vi "Variable list Tool digital.vi"() -> (6 "Variant":variant, 10 "Array":T1[](array[typedef]))   [LabVIEW 2011]
uses:
  Measurments Handling/Fixed Digital Channel Definition.ctl
  Measurments Handling/Update frequensies.ctl
  Measurments Handling/Channel catagory Enum.ctl
  Variable List Tool Digital.ctl
  Measurments Handling/Common/Variable List Common Digital.ctl
  <vilib>/Utility/VariantDataType/GetNumericInfo.vi
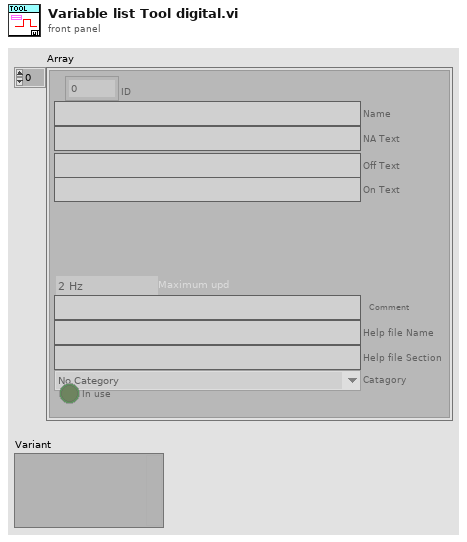
[diagram p1: front panel]
types:
  T1 = typedef "Fixed Digital Channel Definition.ctl" = cluster{"ID":u16, "Name":string, "NA Text":string, "Off Text":string, "On Text":string, "Maximum upd":T2, "Comment":string, "Help file Name":string, "Help file Section ":string, "Catagory":T3, "In use":bool}
  T2 = typedef "Update frequensies.ctl" = enum16{"2 Hz", "1 Hz", "0.1 Hz"}
  T3 = typedef "Channel catagory Enum.ctl" = enum16{"No Category", "Power", "Temperature", "Pressure"}
  T4 = typedef "Variable List Common Digital.ctl" = enum16{"PCP Connected", "PCP PC Control", "HV PSU connected", "HV PSU HV Active", "Modem Connected", "Tool Connected", "CanBus interface"}
  T5 = typedef "Variable List Tool Digital.ctl" = enum16{"Tool Error Controller", "Tool Stopped Controller", "Tool Relay 1", "Tool Relay 2", "Tool Both Relays", "Tool node Pressure 1", "Tool Error Pressure 1", "Tool Stopped Pressure 1", "Tool node Pressure 2", "Tool Error Pressure 2", "Tool Stopped Pressure 2", "Tool node Solenoid", "Tool Error Solenoid", "Tool Stopped Solenoid", "Tool Solenoid 1", "Tool Solenoid 2", "Tool Solenoid 3", "Tool node PSU", "Tool Error PSU", "Tool Stopped PSU", "Upper Tension Sub", "Tool Error Upper Tension Sub", "Tool Stopped Upper Tension Sub", "Lower Tension Sub", "Tool Error Lower Tension Sub", "Tool Stopped Lower Tension Sub", "Stroke Target seeking", "Stroke Moving Out", "Stroke Moving Inn", "Stroke valves set for Out", "Stroke valves set for In", "Stroke In (force)", "Stroke Out (force)", "Stroke Force decreasing(in)", "Stroke Force decreasing(out)", "Stroke Force change not correct", "Stroke SLIPS established P1", "Stroke SLIPS established P2", "Stroke SLIPS established", "Stroke Pressure Monitor Ongoing", "Stroke Pressure Monitor Ending ", "Tool Stroke enable Valve", "Tool Stroke direction Valve", "Tool Anchor Valve", "Stroker Var19 - Reserved", "Stroker Var20 - Reserved", "Stroker Var21 - Reserved", "Stroker Var22 - Reserved", "Stroker Var23 - Reserved", "Stroker Var24 - Reserved", "Tractor Var1 - Reserved", "Tractor Var2 - Reserved", "Tractor Var3 - Reserved", "Tractor Var4 - Reserved", "Tractor Var5 - Reserved", "Tractor Var6 - Reserved", "Tractor Var7 - Reserved", "Tractor Var8 - Reserved", "Oil filling mode", "Mill Bit Direction", "Position control", "Anchor", "Driller Var5 - Reserved", "Driller Var6 - Reserved", "Driller Var7 - Reserved", "Driller Var8 - Reserved"}
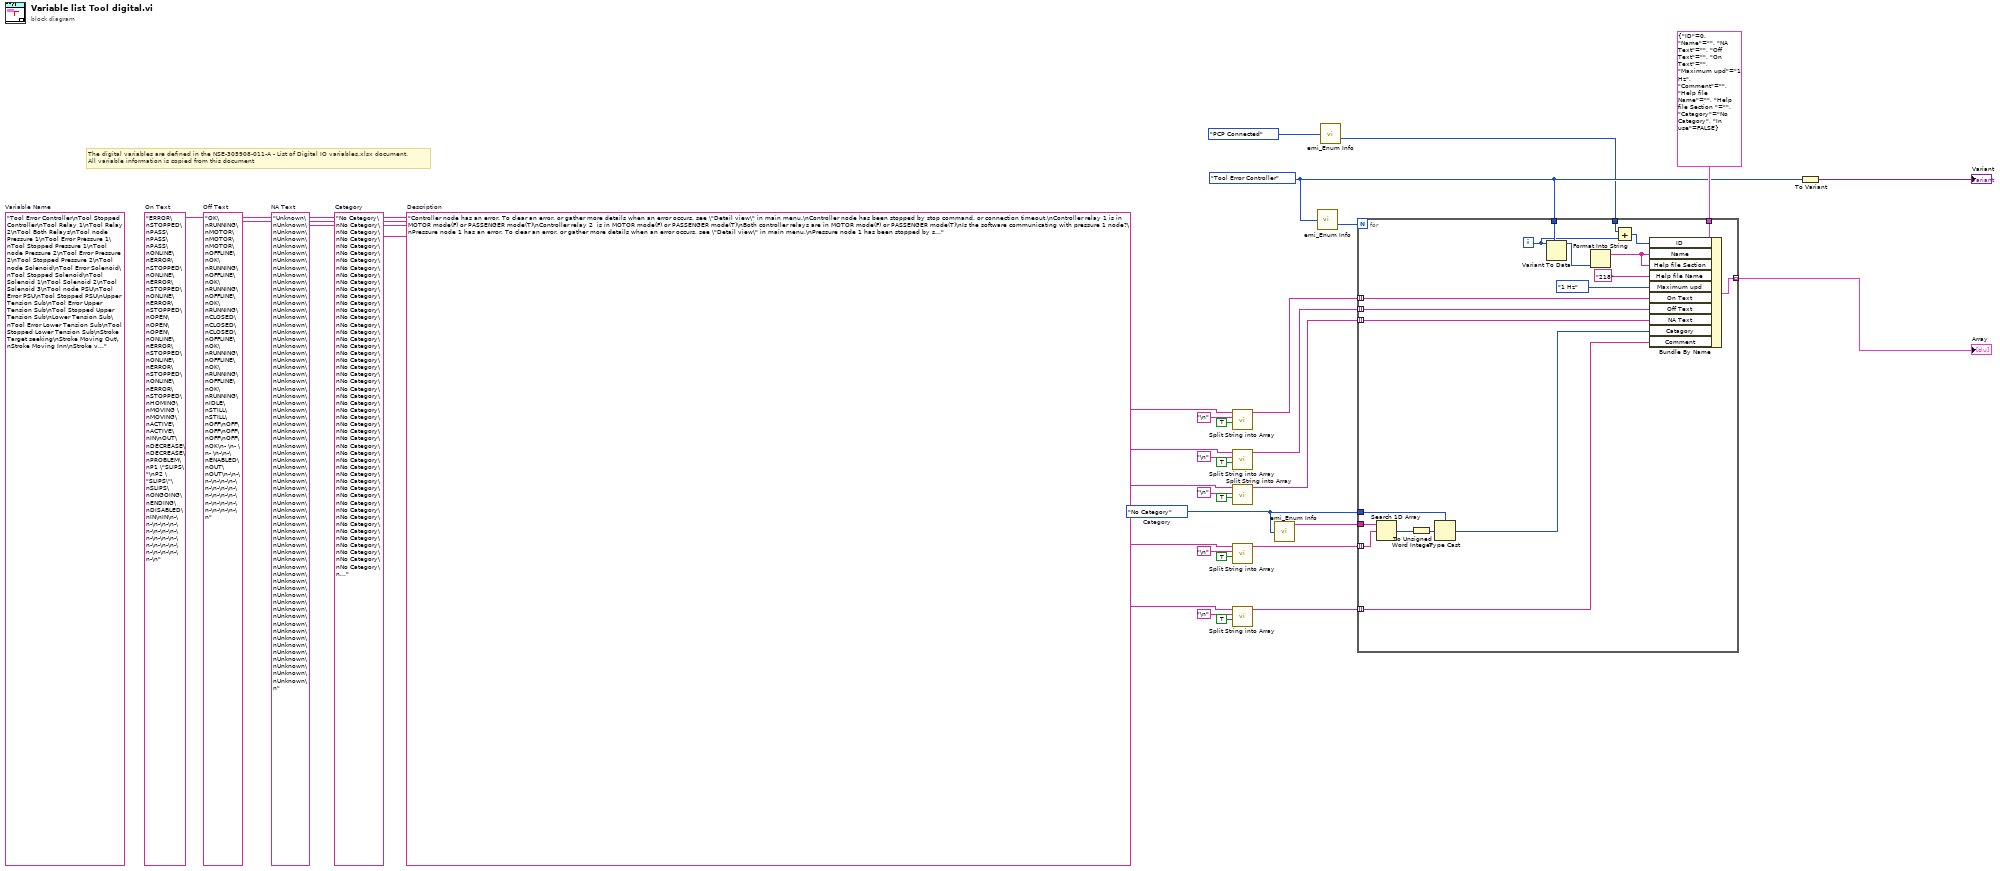
[diagram p0: block diagram]
diagram:
  w3 = Variable_List_Tool_Digital."Tool Error Controller"
  w6 = Channel_catagory_Enum."No Category"  # Category
  w12 = "No Category\nNo Category\nNo Category\nNo Category\nNo Category\nNo Category\nNo Category\nNo Category\nNo Category\nNo Category\nNo Category\nNo Category\nNo Category\nNo Category\nNo Category\nNo Category\nNo Category\nNo Category\nNo Category\nNo Category\nNo Category\nNo Category\nNo Category\nNo Category\nNo Category\nNo Category\nNo Category\nNo Category\nNo Category\nNo Category\nNo Category\nNo Category\nNo Category\nNo Category\nNo Category\nNo Category\nNo Category\nNo Category\nNo Category\nNo Category\nNo Category\nNo Category\nNo Category\nNo Category\nNo Category\nNo Category\nNo Category\nNo Category\nNo Category\nNo Category\nNo Category\nNo Category\nNo Category\nNo Category\nNo Category\nNo Category\nNo Category\nNo Category\nNo Category\nNo Category\nNo Category\nNo Category\nNo Category\nNo Category\nNo Category\nNo Category\n"  # Category
  w4 = "Controller node has an error. To clear an error, or gather more details when an error occurs, see \"Detail view\" in main menu.\nController node has been stopped by stop command, or connection timeout.\nController relay 1 is in MOTOR mode(F) or PASSENGER mode(T)\nController relay 2  is in MOTOR mode(F) or PASSENGER mode(T)\nBoth controller relays are in MOTOR mode(F) or PASSENGER mode(T)\nIs the software communicating with pressure 1 node?\nPressure node 1 has an error. To clear an error, or gather more details when an error occurs, see \"Detail view\" in main menu.\nPressure node 1 has been stopped by stop command, or connection timeout.\nIs the software communicating with pressure 2 node?\nPressure node 2 has an error. To clear an error, or gather more details when an error occurs, see \"Detail view\" in main menu.\nPressure node 2 has been stopped by stop command, or connection timeout.\nIs the software communicating with the solenoid node?\nSolenoid node has an error. To clear an error, or gather more details when an error occurs, see \"Detail view\" in main menu.\nSolenoid node has been stopped by stop command, or connection timeout.\n-\n-\n-\nIs the software communicating with the PSU node?\nPSU node has an error. To clear an error, or gather more details when an error occurs, see \"Detail view\" in main menu.\nPSU node has been stopped by stop command, or connection timeout.\nIs the software communicating with the upper tension sub node.\nUpper Tension Sub node has an error. To clear an error, or gather more details when an error occurs, see \"Detail view\" in main menu.\nUpper Tension Sub node has been stopped by stop command, or connection timeout.\nIs the software communicating with the lower tension sub node.\nLower Tension Sub node has an error. To clear an error, or gather more details when an error occurs, see \"Detail view\" in main menu.\nLower Tension Sub node has been stopped by stop command, or connection timeout.\nTool stroke is moving to a preset mm target. This should be the result of a \"Go to\" command. \nStroke has been detected as moving out based on position data over time\nStroke has been detected as moving in based on position data over time\nStroke hydraulic valves are positioned to move the stroke out.\nStroke hydraulic valves are positioned to move the stroke in.\nPressure readings are indicating that the stroke is moving in\nPressure readings are indicating that the stroke is moving out\nPressure readings are indicating that the inward stroke force is decreasing. \nPressure readings are indicating that the outward stroke force is decreasing. \nStroke force is decreasing when it should be increasing. Expected: When pressure is over limit to indicate movement, and valves are set for movement, the pressure on the stroking side is not expected to decrease.\nPressure node 1 indicates that SLIPS has been established.\nPressure node 2 indicates that SLIPS has been established.\nBoth pressure nodes indicate that SLIPS has been established.\nPressure monitoring state.\nPressure monitoring shutting down. Should never be active for long periods.\nStroke enable solenoid open(F) or closed(T)\nStroke direction solenoid open(F) or closed(T)\nAnchor solenoid open(F) or closed(T)\n-\n-\n-\n-\n-\n-\n-\n-\n-\n-\n-\n-\n-\n-\n-\n-\n-\n-\n-\n-\n-\n-\n"  # Description
  w17 = "Unknown\nUnknown\nUnknown\nUnknown\nUnknown\nUnknown\nUnknown\nUnknown\nUnknown\nUnknown\nUnknown\nUnknown\nUnknown\nUnknown\nUnknown\nUnknown\nUnknown\nUnknown\nUnknown\nUnknown\nUnknown\nUnknown\nUnknown\nUnknown\nUnknown\nUnknown\nUnknown\nUnknown\nUnknown\nUnknown\nUnknown\nUnknown\nUnknown\nUnknown\nUnknown\nUnknown\nUnknown\nUnknown\nUnknown\nUnknown\nUnknown\nUnknown\nUnknown\nUnknown\nUnknown\nUnknown\nUnknown\nUnknown\nUnknown\nUnknown\nUnknown\nUnknown\nUnknown\nUnknown\nUnknown\nUnknown\nUnknown\nUnknown\nUnknown\nUnknown\nUnknown\nUnknown\nUnknown\nUnknown\nUnknown\nUnknown\n"  # NA Text
  w20 = "OK\nRUNNING\nMOTOR\nMOTOR\nMOTOR\nOFFLINE\nOK\nRUNNING\nOFFLINE\nOK\nRUNNING\nOFFLINE\nOK\nRUNNING\nCLOSED\nCLOSED\nCLOSED\nOFFLINE\nOK\nRUNNING\nOFFLINE\nOK\nRUNNING\nOFFLINE\nOK\nRUNNING\nIDLE\nSTILL\nSTILL\nOFF\nOFF\nOFF\nOFF\nOFF\nOFF\nOK\n- \n- \n- \n-\n-\nENABLED\nOUT\nOUT\n-\n-\n-\n-\n-\n-\n-\n-\n-\n-\n-\n-\n-\n-\n-\n-\n-\n-\n-\n-\n-\n-\n"  # Off Text
  w23 = "ERROR\nSTOPPED\nPASS\nPASS\nPASS\nONLINE\nERROR\nSTOPPED\nONLINE\nERROR\nSTOPPED\nONLINE\nERROR\nSTOPPED\nOPEN\nOPEN\nOPEN\nONLINE\nERROR\nSTOPPED\nONLINE\nERROR\nSTOPPED\nONLINE\nERROR\nSTOPPED\nHOMING\nMOVING \nMOVING\nACTIVE\nACTIVE\nIN\nOUT\nDECREASE\nDECREASE\nPROBLEM\nP1 \"SLIPS\"\nP2 \"SLIPS\"\nSLIPS\nONGOING\nENDING\nDISABLED\nIN\nIN\n-\n-\n-\n-\n-\n-\n-\n-\n-\n-\n-\n-\n-\n-\n-\n-\n-\n-\n-\n-\n-\n-\n"  # On Text
  (unwired) "Tool Error Controller\nTool Stopped Controller\nTool Relay 1\nTool Relay 2\nTool Both Relays\nTool node Pressure 1\nTool Error Pressure 1\nTool Stopped Pressure 1\nTool node Pressure 2\nTool Error Pressure 2\nTool Stopped Pressure 2\nTool node Solenoid\nTool Error Solenoid\nTool Stopped Solenoid\nTool Solenoid 1\nTool Solenoid 2\nTool Solenoid 3\nTool node PSU\nTool Error PSU\nTool Stopped PSU\nUpper Tension Sub\nTool Error Upper Tension Sub\nTool Stopped Upper Tension Sub\nLower Tension Sub\nTool Error Lower Tension Sub\nTool Stopped Lower Tension Sub\nStroke Target seeking\nStroke Moving Out\nStroke Moving Inn\nStroke valves set for Out\nStroke valves set for In\nStroke In (force)\nStroke Out (force)\nStroke Force decreasing(in)\nStroke Force decreasing(out)\nStroke Force change not correct\nStroke SLIPS established P1\nStroke SLIPS established P2\nStroke SLIPS established\nStroke Pressure Monitor Ongoing\nStroke Pressure Monitor Ending \nTool Stroke enable Valve\nTool Stroke direction Valve\nTool Anchor Valve\nStroker Var19 - Reserved\nStroker Var20 - Reserved\nStroker Var21 - Reserved\nStroker Var22 - Reserved\nStroker Var23 - Reserved\nStroker Var24 - Reserved\nTractor Var1 - Reserved\nTractor Var2 - Reserved\nTractor Var3 - Reserved\nTractor Var4 - Reserved\nTractor Var5 - Reserved\nTractor Var6 - Reserved\nTractor Var7 - Reserved\nTractor Var8 - Reserved\nOil filling mode\nMill Bit Direction\nPosition control\nAnchor\nDriller Var5 - Reserved\nDriller Var6 - Reserved\nDriller Var7 - Reserved\nDriller Var8 - Reserved\n"  # Variable Name
  # "The digital variables are defined in the NSE-305908-011-A - List of Digital IO variables.xlsx document.\nAll variable information is copied from this document"
  n1 = call "Split String into Array.vi"("Remove Last Row"=TRUE, "Separator"="\n", "Input string"=w23) -> ("Array of cells"=w11:string[])  [unwired: 8 in]
  n2 = call "Split String into Array.vi"("Remove Last Row"=TRUE, "Separator"="\n", "Input string"=w20) -> ("Array of cells"=w10:string[])  [unwired: 8 in]
  n3 = call "Split String into Array.vi"("Remove Last Row"=TRUE, "Separator"="\n", "Input string"=w17) -> ("Array of cells"=w9:string[])  [unwired: 8 in]
  n4 = call "Split String into Array.vi"("Remove Last Row"=TRUE, "Separator"="\n", "Input string"=w12) -> ("Array of cells"=w8:string[])  [unwired: 8 in]
  n5 = call "Split String into Array.vi"("Remove Last Row"=TRUE, "Separator"="\n", "Input string"=w4) -> ("Array of cells"=w5:string[])  [unwired: 8 in]
  n6 = call "emi_Enum Info.vi"("Enum"=w6) -> ("Text Elements"=w7:string[])  [unwired: 11 in, 3 out]
  n7 = call "emi_Enum Info.vi"("Enum"=w3) -> ("Numb Elements"=w27:i32)  [unwired: 11 in, 3 out]
  n8 = call "emi_Enum Info.vi"("Enum"=Variable_List_Common_Digital."PCP Connected" ("Action")) -> ("Numb Elements"=w1:i32)  [unwired: 11 in, 3 out]
  n9 = for {
    N: w27 -> [_]
    tunnel: w3 -> [w33]
    tunnel: T1 {"ID"=0, "Name"="", "NA Text"="", "Off Text"="", "On Text"="", "Maximum upd"=enum."1 Hz", "Comment"="", "Help file Name"="", "Help file Section "="", "Catagory"=enum."No Category", "In use"=FALSE} ("Variable Defenition") -> [w47]
    tunnel: [w48] -> w28 mode=indexing
    tunnel: w11 -> [w43] mode=indexing
    tunnel: w10 -> [w42] mode=indexing
    tunnel: w9 -> [w41] mode=indexing
    tunnel: w8 -> [w38] mode=indexing
    tunnel: w7 -> [w37]
    tunnel: w6 -> [w36]
    tunnel: w5 -> [w34] mode=indexing
    tunnel: w1 -> [w32]
    i -> [w30]
    n10 = Search 1D Array(1D array=w37, element=w38) -> (index of element=w40:i32)  [unwired: 1 in]
    n11 = To Unsigned Word Integer(number=w40) -> (unsigned 16bit integer=w39:u16)
    n12 = Type Cast(type=w36, x=w39) -> (*(type *) &x=w35:T3)
    n13 = Variant To Data(type=w33, Variant=w30) -> (data=w49:T5)  [unwired: 1 in, 1 out]
    n14 = Format Into String(w49) -> (resulting string=w46:string)  [unwired: 3 in, 1 out]
    n15 = Add(x=w32, y=w30) -> (x+y=w31:i32)
    n16 = Bundle By Name(cluster=w47, "ID"=w31, "Name"=w46, "Help file Section"=w46, "Help file Name"="218", "Maximum upd"=Update_frequensies."1 Hz", "On Text"=w43, "Off Text"=w42, "NA Text"=w41, "Catagory"=w35, "Comment"=w34) -> (w48:T1)
  }
  "Array" <- w28
  n17 = To Variant(anything=w3) -> (Variant=→"Variant":variant)
